vi "Enable MPG.vi"(8 "error in":errorcluster, 11 "Gantry in":refnum<class "Gantry.lvclass">) -> (0 "error out":errorcluster, 3 "Gantry out":refnum<class "Gantry.lvclass">)   [LabVIEW 2026, in "Gantry.lvclass"]
uses:
  Gantry.lvclass
  FlexWorktable/FlexWorktable.lvclass
  <instrlib>/Aerotech Automation1/Aerotech Automation1.lvlib
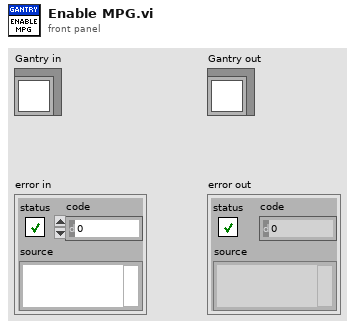
[diagram p1: front panel]
types:
  T1 = enum16{"open", "replace", "create", "open or create", "replace or create", "replace or create with confirmation"}
  T2 = typedef "Virtual Modes.ctl" = enum16{"Nonvirtual", "Virtual"}
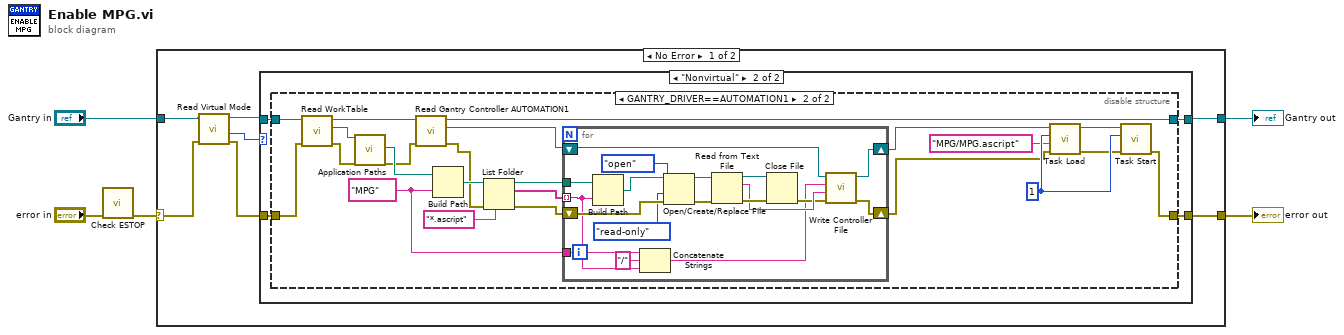
[diagram p0: block diagram]
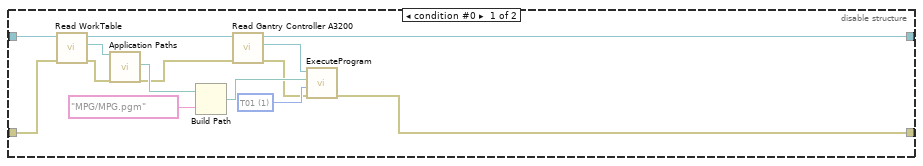
[diagram p3: hidden frame]
diagram:
  n1 = call "Check ESTOP.vi"("error in"="error in") -> ("error out"=w2:errorcluster)  [unwired: 10 in]
  n2 = case shown="No Error" w2 {
    selector: w2 -> [w8 w75]
    tunnel: [w11 w75] -> w5
    tunnel: [w12 w74] -> w4
    tunnel: "Gantry in" -> [w10 w74]
    frame No Error {
      n3 = call-dynamic "Read Virtual Mode.vi"("error in (no error)"=w8, "Gantry in"=w10) -> ("error out"=w7:errorcluster, "Virtual Mode"=w6:T2, "Gantry out"=w9:refnum<class "Gantry.lvclass">)  [unwired: 6 in, 1 out]
      n4 = case shown="\"Nonvirtual\"" w6 {
        tunnel: w7 -> [w13 w16]
        tunnel: [w14 w15] -> w12
        tunnel: [w13 w18] -> w11
        tunnel: w9 -> [w14 w17]
        frame "Virtual" {
        }
        frame "Nonvirtual" {
          n5 = disable-structure shown="GANTRY_DRIVER==AUTOMATION1" {
            disable-tunnel: [w29 w47] -> w18
            disable-tunnel: w17 -> [w28 w45]
            disable-tunnel: w16 -> [w24 w44]
            disable-tunnel: [w21 w46] -> w15
            frame condition #0 {
              w32 = 1 items=["TLibrary", "T01", "T02", "T03", "T04", "T05", "T06", "T07", "T08", "T09", "T10", "T11", "T12", "T13", "T14", "T15", "T16", "T17", "T18", "T19", "T20", "T21", "T22", "T23", "T24", "T25", "T26", "T27", "T28", "T29", "T30", "T31"] ("taskId")
              n6 = call-dynamic "Read WorkTable.vi"("error in"=w24, "Gantry Class in"=w28) -> ("error out"=w25:errorcluster, "Worktable"=w27:refnum<class "FlexWorktable.lvclass">, "Gantry Class out"=w23:refnum<class "Gantry.lvclass">)  [unwired: 7 in]
              n7 = call "Application Paths.vi"("FlexWorktable in"=w27, "error in (no error)"=w25) -> ("Config Path"=w26:path, "error out"=w22:errorcluster)  [unwired: 11 in, 5 out]
              n8 = Build Path(base path=w26, name or relative path="MPG/MPG.pgm") -> (appended path=w30:path)
              n9 = call "Read Gantry Controller A3200.vi"("error in (no error)"=w22, "Gantry in"=w23) -> ("error out"=w20:errorcluster, "A3200 controller out"=w19:refnum<k24>, "Gantry out"=w21:refnum<class "Gantry.lvclass">)  [unwired: 7 in]
              n10 = call "ExecuteProgram.vi"("error in (no error)"=w20, "taskId"=w32, "program name and path"=w30, "controller in"=w19) -> ("error out"=w29:errorcluster)  [unwired: 5 in, 2 out]
            }
            frame condition #1 (active) {
              w49 = 1 ("Task Index")
              w35 = "MPG"
              n11 = call-dynamic "Read WorkTable.vi"("error in"=w44, "Gantry Class in"=w45) -> ("error out"=w53:errorcluster, "Worktable"=w55:refnum<class "FlexWorktable.lvclass">, "Gantry Class out"=w52:refnum<class "Gantry.lvclass">)  [unwired: 7 in]
              n12 = call "Application Paths.vi"("FlexWorktable in"=w55, "error in (no error)"=w53) -> ("Config Path"=w54:path, "error out"=w51:errorcluster)  [unwired: 11 in, 5 out]
              n13 = call "Read Gantry Controller AUTOMATION1.vi"("error in (no error)"=w51, "Gantry in"=w52) -> ("error out"=w41:errorcluster, "Controller AUTOMATION1"=w39:refnum<k24>, "Gantry out"=w46:refnum<class "Gantry.lvclass">)  [unwired: 7 in]
              n14 = Build Path(base path=w54, name or relative path=w35) -> (appended path=w42:path)
              n15 = List Folder(path=w42, pattern="*.ascript", error in=w41) -> (path out=w38:path, filenames=w37:string[], error out=w36:errorcluster)  [unwired: 1 in, 1 out]
              n16 = for {
                tunnel: w38 -> [w73]
                tunnel: w37 -> [w57] mode=indexing
                shift-right: [w61] -> w34
                shift-left: w39 -> [w62]
                shift-right: [w60] -> w33
                shift-left: w36 -> [w71]
                tunnel: w35 -> [w59]
                n17 = Build Path(base path=w73, name or relative path=w57) -> (appended path=w72:path)
                n18 = Concatenate Strings(w59, "/" ("string"), w57) -> (w58:string)
                n19 = Open/Create/Replace File(file path (use dialog)=w72, error in=w71, operation (0:open)=T1."open", access (0:read/write)=enum16{"read/write", "read-only", "write-only"}."read-only") -> (refnum out=w67:refnum<file>, error out=w68:errorcluster)  [unwired: 2 in, 1 out]
                n20 = Read from Text File(file (use dialog)=w67, error in=w68) -> (refnum out=w65:refnum<file>, text=w64:string, error out=w66:errorcluster)  [unwired: 2 in, 1 out]
                n21 = Close File(refnum=w65, error in=w66) -> (error out=w63:errorcluster)  [unwired: 1 out]
                n22 = call <instrlib>:"Write Controller File.vi"("error in (no error)"=w63, "File Contents"=w64, "controllerFileName"=w58, "Controller Refnum in"=w62) -> ("error out"=w60:errorcluster, "Controller Refnum out"=w61:refnum<k24>)  [unwired: 6 in]
              }
              n23 = call <instrlib>:"Task Load.vi"("error in (no error)"=w33, "Controller Filename"="MPG/MPG.ascript", "Task Index"=w49, "Controller Refnum"=w34) -> ("error out"=w48:errorcluster, "Controller Refnum out"=w50:refnum<k24>)  [unwired: 6 in]
              n24 = call <instrlib>:"Task Start.vi"("error in (no error)"=w48, "Task Index"=w49, "Controller Refnum"=w50) -> ("error out"=w47:errorcluster)  [unwired: 7 in, 1 out]
            }
          }
        }
      }
    }
    frame Error {
    }
  }
  "error out" <- w5
  "Gantry out" <- w4
